vi "Set Camera Mode Message to JSON.vi"(2 "error in":errorcluster, 3 "Set Camera Mode Message":T1={"type"="camera_mode", "Vision Mode"={"message"="vision", "Active?"=TRUE}, "Intake Mode"={"message"="intake", "Active?"=FALSE}}) -> (0 "error out":errorcluster, 1 "JSON string":string)   [LabVIEW 2016]
uses:
  Set Camera Mode Message.ctl
  Generic Message.ctl
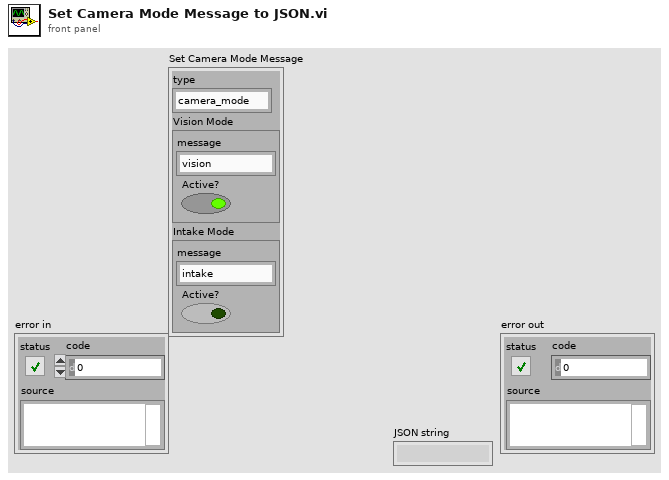
[diagram p1: front panel]
types:
  T1 = typedef "Set Camera Mode Message.ctl" = cluster{"type":string, "Vision Mode":cluster{"message":string, "Active?":bool}, "Intake Mode":cluster{"message":string, "Active?":bool}}
  T2 = typedef "Generic Message.ctl" = cluster{"type":string, "message":string}
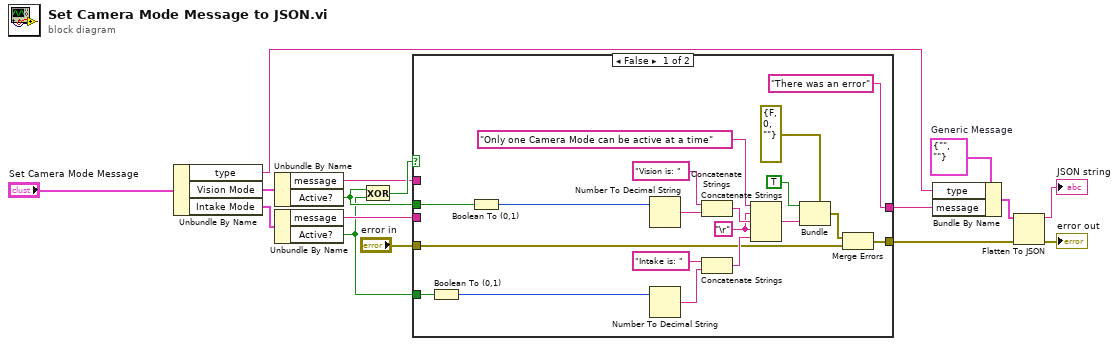
[diagram p0: block diagram]
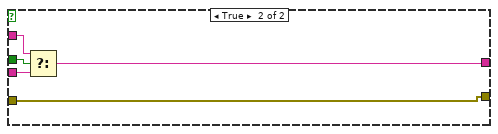
[diagram p2: hidden frame]
diagram:
  w1 = T2 {"type"="", "message"=""}  # Generic Message
  n1 = Unbundle By Name("Set Camera Mode Message") -> ("type"=w5:string, "Vision Mode"=w14:cluster{"message":string, "Active?":bool}, "Intake Mode"=w13:cluster{"message":string, "Active?":bool})
  n2 = Unbundle By Name(w14) -> ("message"=w10:string, "Active?"=w11:bool)
  n3 = Unbundle By Name(w13) -> ("message"=w9:string, "Active?"=w8:bool)
  n4 = Exclusive Or(1:w8, 2:w11) -> (0:w12:bool)
  n5 = case shown="False" w12 {
    tunnel: w11 -> [w31 w40]
    tunnel: w10 -> [_ w39]
    tunnel: w9 -> [_ w38]
    tunnel: ["There was an error" ("Message") w37] -> w4
    tunnel: w8 -> [w24 _]
    tunnel: "error in" -> [w19 w36]
    tunnel: [w18 w36] -> w6
    frame False {
      w28 = "\r"
      n6 = Boolean To (0,1)(Boolean=w24) -> (0, 1=w25:i16)
      n7 = Boolean To (0,1)(Boolean=w31) -> (0, 1=w30:i16)
      n8 = Number To Decimal String(number=w30) -> (decimal integer string=w27:string)  [unwired: 1 in]
      n9 = Number To Decimal String(number=w25) -> (decimal integer string=w23:string)  [unwired: 1 in]
      n10 = Concatenate Strings("Vision is: " ("string"), w27) -> (w29:string)
      n11 = Concatenate Strings("Intake is: " ("string"), w23) -> (w22:string)
      n12 = Concatenate Strings("Only one Camera Mode can be active at a time" ("source"), w28, w29, w28, w22) -> (w21:string)
      n13 = Bundle(cluster=errorcluster {"status"=FALSE, "code"=0, "source"=""} ("error constant"), "status"=TRUE, "source"=w21) -> (w20:errorcluster)  [unwired: 1 in]
      n14 = Merge Errors(w20, w19) -> (w18:errorcluster)
    }
    frame True {
      n15 = Select(t=w39, s=w40, f=w38) -> (s? t:f=w37:string)
    }
  }
  n16 = Bundle By Name(cluster=w1, "type"=w5, "message"=w4) -> (w3:T2)
  n17 = Flatten To JSON(anything=w3, error in (no error)=w6) -> (JSON string=→"JSON string":string, 11:→"error out":errorcluster)  [unwired: 1 in]
